vi "Get Wheel Parameters.vi"(8 "error in (no error)":errorcluster, 11 "wheel in":refnum<class "NI_Robotics_Wheel.lvclass">) -> (0 "error out":errorcluster, 1 "wheel name":string, 2 "wheel parameters":T1={"wheel radius"=1.0, "gear ratio"=1.0, "forward rotation direction"=0} {"forward rotation direction" items=["Clockwise", "Counterclockwise"]}, 3 "wheel out":refnum<class "NI_Robotics_Wheel.lvclass">)   [LabVIEW 2017, in "NI_Robotics_Wheel.lvclass"]
uses:
  <vilib>/robotics/Steering/Wheel/NI_Robotics_Wheel.lvclass
  <vilib>/robotics/Steering/Wheel/Wheel Parameters.ctl
  <vilib>/robotics/Steering/Wheel/Rotation Direction.ctl
  <vilib>/robotics/Steering/Wheel/NI_Robotics_Wheel.lvclass/NI_Robotics_Wheel.ctl
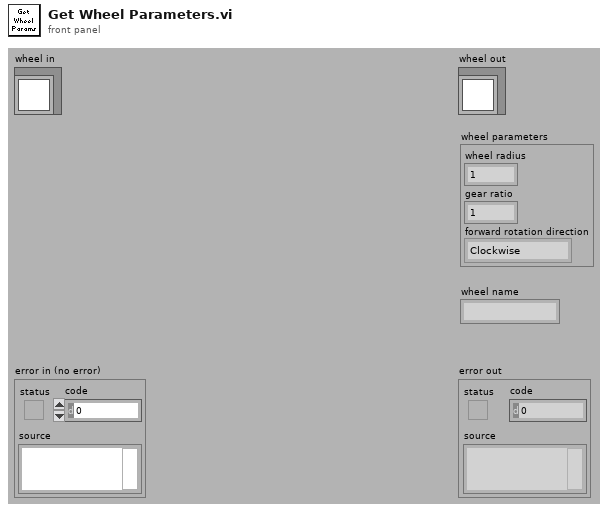
[diagram p1: front panel]
types:
  T1 = typedef "NI_Robotics_Wheel.lvclass/Wheel Parameters.ctl" = cluster{"wheel radius":dbl, "gear ratio":dbl, "forward rotation direction":T2}
  T2 = typedef "NI_Robotics_Wheel.lvclass/Rotation Direction.ctl" = u16
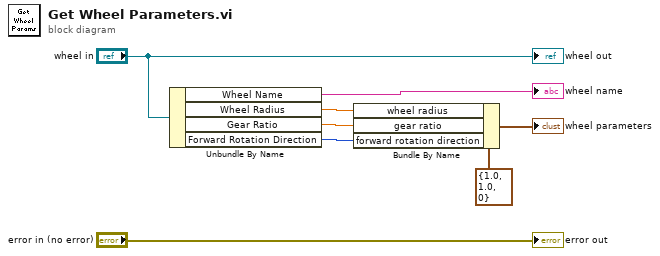
[diagram p0: block diagram]
diagram:
  n1 = Unbundle By Name("wheel in") -> ("Wheel Name"=→"wheel name":string, "Wheel Radius"=w3:dbl, "Gear Ratio"=w2:dbl, "Forward Rotation Direction"=w1:T2)
  n2 = Bundle By Name(cluster=T1 {"wheel radius"=1.0, "gear ratio"=1.0, "forward rotation direction"=0} ("wheel parameters"), "wheel radius"=w3, "gear ratio"=w2, "forward rotation direction"=w1) -> (→"wheel parameters":T1)
  "error out" <- "error in (no error)"
  "wheel out" <- "wheel in"
